vi "sub-Language dir.vi"() -> (0 "folder":path)   [LabVIEW 2011]
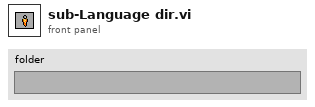
[diagram p1: front panel]
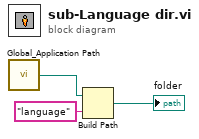
[diagram p0: block diagram]
diagram:
  n1 = call "Global_Application Path.vi"() -> ("程序路径"=w3:path)  [unwired: 1 in]
  n2 = Build Path(base path=w3, name or relative path="language" ("名称或相对路径")) -> (appended path=→"folder":path)
